vi "MDAQ_GraphHelper.vi"(7 "Concurrent CV Arrays":T2, 9 "Normalised":bool, 10 "Input Cluster":T4 {"CV"."Temperature Array" scale=0.0..100.0}, 11 "Amplitude Plot":refnum<vi>) -> (1 "To Temp Graph":T1(array[cluster]), 2 "To Graph":T3(array[cluster]), 3 "Array":cluster{"Numeric":dbl, dbl}[](array[cluster]))   [LabVIEW 2021]
uses:
  GUI_Def.ctl
  Mode_Enum.ctl
  Array_Cluster.ctl
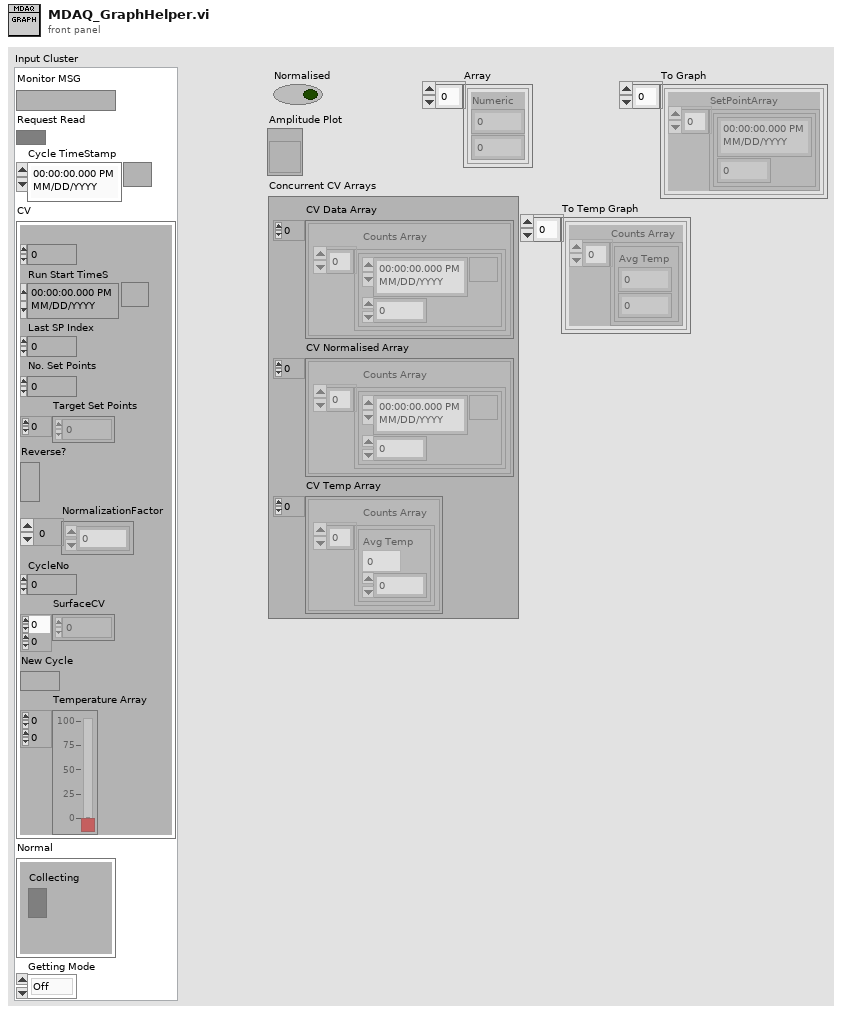
[diagram p1: front panel]
types:
  T1 = cluster{"Counts Array":cluster{"Avg Temp":dbl, dbl}[]}[]
  T2 = typedef "Array_Cluster.ctl" = cluster{"CV Data Array":cluster{"Counts Array":cluster{timestamp, i32}[]}[], "CV Normalised Array":cluster{"Counts Array":cluster{timestamp, dbl}[]}[], "CV Temp Array":cluster{"Counts Array":cluster{"Avg Temp":dbl, dbl}[]}[]}
  T3 = cluster{"SetPointArray":cluster{timestamp, dbl}[]}[]
  T4 = typedef "GUI_Def.ctl" = cluster{"Monitor MSG":string, "Request Read":bool, "Cycle TimeStamp":timestamp, "CV":cluster{"Set Point Index":u32, "Run Start TimeS":timestamp, "Last SP Index":u32, "No. Set Points":u32, "Target Set Points":i32[], "Reverse?":bool, "NormalizationFactor":i32[], "CycleNo":i32, "SurfaceCV":dbl[][], "New Cycle":bool, "Temperature Array":dbl[][]}, "Normal":cluster{"Collecting":bool}, "Getting Mode":T5}
  T5 = typedef "Mode_Enum.ctl" = enum16{"Off", "Normal", "CV+Temp", "CV"}
  T6 = cluster{"Counts Array":cluster{timestamp, dbl}[]}[]
  T7 = cluster{"Counts Array":cluster{timestamp, i32}[]}[]
  T8 = cluster{"BackgroundArray":cluster{timestamp, i32}[]}[]
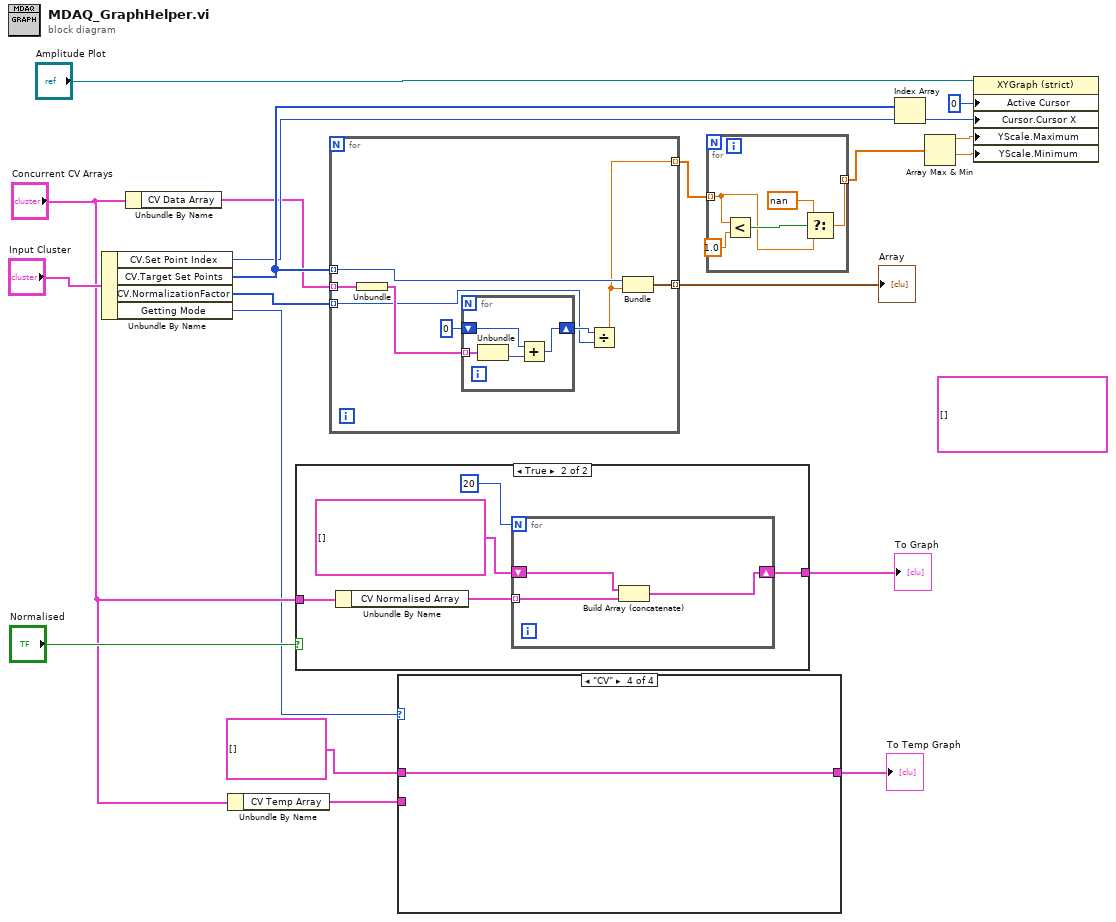
[diagram p0: block diagram]
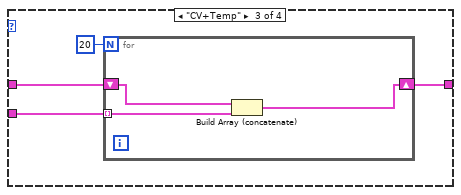
[diagram p4: hidden frame]
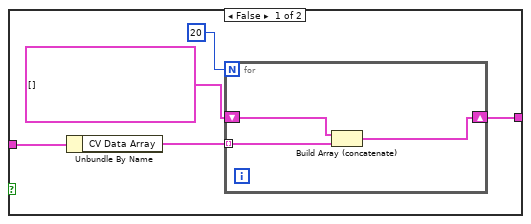
[diagram p5: hidden frame]
diagram:
  (unwired) T6 []
  n1 = Unbundle By Name("Input Cluster") -> ("CV.Set Point Index"=w13:u32, "CV.Target Set Points"=w14:i32[], "CV.NormalizationFactor"=w17:i32[], "Getting Mode"=w1:T5)
  n2 = Unbundle By Name("Concurrent CV Arrays") -> ("CV Data Array"=w6:T7)
  n3 = Unbundle By Name("Concurrent CV Arrays") -> ("CV Temp Array"=w4:T1)
  n4 = case shown="True" "Normalised" {
    tunnel: "Concurrent CV Arrays" -> [w24 w32]
    tunnel: [w22 w31] -> w19
    frame False {
      n5 = Unbundle By Name(w24) -> ("CV Data Array"=w25:T7)
      n6 = for {
        N: 20 -> [_]
        tunnel: w25 -> [w28] mode=indexing
        shift-right: [w27] -> w22
        shift-left: T8 [] -> [w26]
        n7 = Build Array (concatenate)(w26, w28) -> (w27:T7)
      }
    }
    frame True {
      n8 = Unbundle By Name(w32) -> ("CV Normalised Array"=w33:T6)
      n9 = for {
        N: 20 -> [_]
        tunnel: w33 -> [w36] mode=indexing
        shift-right: [w35] -> w31
        shift-left: T6 [] -> [w34]
        n10 = Build Array (concatenate)(w34, w36) -> (w35:T6)
      }
    }
  }
  "To Graph" <- w19
  n11 = for {
    tunnel: w14 -> [w44] mode=indexing
    tunnel: w6 -> [w43] mode=indexing
    tunnel: [w40] -> w11 mode=indexing
    tunnel: w17 -> [w38] mode=indexing
    tunnel: [w37] -> w8 mode=indexing
    n12 = Unbundle(w43) -> ("Counts Array"=w42:cluster{timestamp, i32}[])
    n13 = for {
      tunnel: w42 -> [w48] mode=indexing
      shift-right: [w47] -> w39
      shift-left: 0 -> [w45]
      n14 = Unbundle(w48) -> (w46:i32)  [unwired: 1 out]
      n15 = Add(x=w45, y=w46) -> (x+y=w47:i32)
    }
    n16 = Divide(x=w39, y=w38) -> (x/y=w37:dbl)
    n17 = Bundle("Numeric"=w44, w37) -> (w40:cluster{"Numeric":i32, dbl})  [unwired: 1 in]
  }
  "Array" <- w11
  n18 = case shown="\"CV\"" w1 {
    tunnel: w4 -> [_ _ w53 _]
    tunnel: T1 [] ("CV Temp Array") -> [w49 w50 w52 w58]
    tunnel: [w49 w50 w51 w58] -> w2
    frame "Off", Default {
    }
    frame "Normal" {
    }
    frame "CV+Temp" {
      n19 = for {
        N: 20 -> [_]
        tunnel: w53 -> [w56] mode=indexing
        shift-right: [w55] -> w51
        shift-left: w52 -> [w57]
        n20 = Build Array (concatenate)(w57, w56) -> (w55:T1)
      }
    }
    frame "CV" {
    }
  }
  "To Temp Graph" <- w2
  n21 = for {
    tunnel: w8 -> [w61] mode=indexing
    tunnel: [w59] -> w7 mode=indexing
    n22 = Less?(x=w61, y=1.0) -> (x < y?=w62:bool)
    n23 = Select(t=nan, s=w62, f=w61) -> (s? t:f=w59:dbl)
  }
  n24 = Index Array(array=w14, index=w13) -> (element=w12:i32)
  n25 = Array Max & Min(array=w7) -> (max value=w10:dbl, min value=w9:dbl)  [unwired: 2 out]
  n26 = property class="XYGraph (strict)"(reference="Amplitude Plot", "Active Cursor"=u32 0, "Cursor.Cursor X"=w12, "YScale.Maximum"=w10, "YScale.Minimum"=w9) -> ()  [unwired: 1 in, 2 out]
